vi "Autonomous Independent.vi"() -> ()   [LabVIEW 2015]
doc: "This VI is called when autonomous begins, and will automatically be terminated when autonomous ends. You can carry out timed or sensor driven robot movement independently without needing to return to the caller."
uses:
  <vilib>/Rock Robotics/Network Tables/NT Read String.vi
  <vilib>/Rock Robotics/WPI/Utilities/WPI_GetSetVariantRefNum.vi
  <vilib>/Rock Robotics/WPI/RobotDrive/WPI_RobotDriveArcadeDrive_Standard(NoSaturation).vi
  <vilib>/Rock Robotics/Network Tables/NT Write Numeric Array.vi
  <vilib>/Rock Robotics/Network Tables/NT Read Number.vi
  Robot Global Data.vi
  <vilib>/Rock Robotics/Network Tables/NT Write Boolean.vi
panel:
  out "Current Movement, for debugging":T1 {"Y Joystick Value" scale=1.0..-1.0; "X Joystick Value" scale=-1.0..1.0}
  in  "Array of robot movements":T2(array[cluster])=[{"X Joystick Value"=0.39393939393939403, "Y Joystick Value"=0.0, "Delay (sec)"=1.0, "Movement Name"="turn"}, {"X Joystick Value"=-0.3737373737373737, "Y Joystick Value"=0.0, "Delay (sec)"=1.0, "Movement Name"="turn back"}] {"Y Joystick Value" scale=1.0..-1.0; "X Joystick Value" scale=-1.0..1.0}
  # "Be sure to right-click and choose Data Operations>>Make Current Value default if you want to save the array values with the VI"
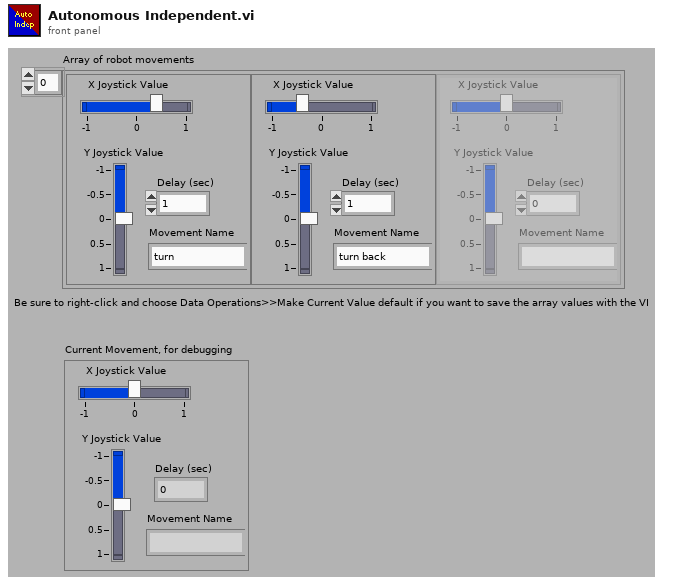
[diagram p1: front panel]
types:
  T1 = cluster{"X Joystick Value":dbl, "Y Joystick Value":dbl, "Delay (sec)":dbl, "Movement Name":string}
  T2 = cluster{"X Joystick Value":dbl, "Y Joystick Value":dbl, "Delay (sec)":dbl, "Movement Name":string}[]
  T3 = typedef "WPI_RobotDriveDevRef.ctl" = cluster{"DevStatus":errorcluster, "Motors[]":T4[], "Square Inputs":bool, "Max Output":dbl}
  T4 = typedef "WPI_MotorControlDeviceRef.ctl" = cluster{"DeviceStatus":errorcluster, "Type":T5, "PWM":cluster{"PWM Channel":T6, "DeadBand":T7}, "CAN":cluster{"Device Number":u8, "Control Mode":T8, "Semaphore":T9, "Max Vout":dbl, "TalonSRX Control Mode":T10}, "Invert":bool}
  T5 = typedef "WPI_MotorControlType.ctl" = enum16{"PWM", "CAN", "CANTalonSRX"}
  T6 = typedef "FPGA_DIOPWMChannel.ctl" = enum8{"PWM 0", "PWM 1", "PWM 2", "PWM 3", "PWM 4", "PWM 5", "PWM 6", "PWM 7", "PWM 8", "PWM 9", "PWM MXP 0", "PWM MXP 1", "PWM MXP 2", "PWM MXP 3", "PWM MXP 4", "PWM MXP 5", "PWM MXP 6", "PWM MXP 7", "PWM MXP 8", "PWM MXP 9", "Invalid"}
  T7 = typedef "WPI_PWMDeadband.ctl" = cluster{"Name":string, "maxPositivePwm":i32, "minPositivePwm":i32, "centerPwm":i32, "maxNegativePwm":i32, "minNegativePwm":i32, "angularRange":u16}
  T8 = typedef "WPI_CANJaguar_ControlMode.ctl" = enum8{"Percent VBus", "Current", "Speed", "Position", "Voltage"}
  T9 = typedef "Semaphore RefNum" = refnum<k1>
  T10 = typedef "WPI_CANTalonSRX_APIControlMode.ctl" = enum8{"Percent VBus", "Speed", "Position", "Slave", "Unchanged / Invalid", "Voltage Compensation", "Current", "Motion Profile"}
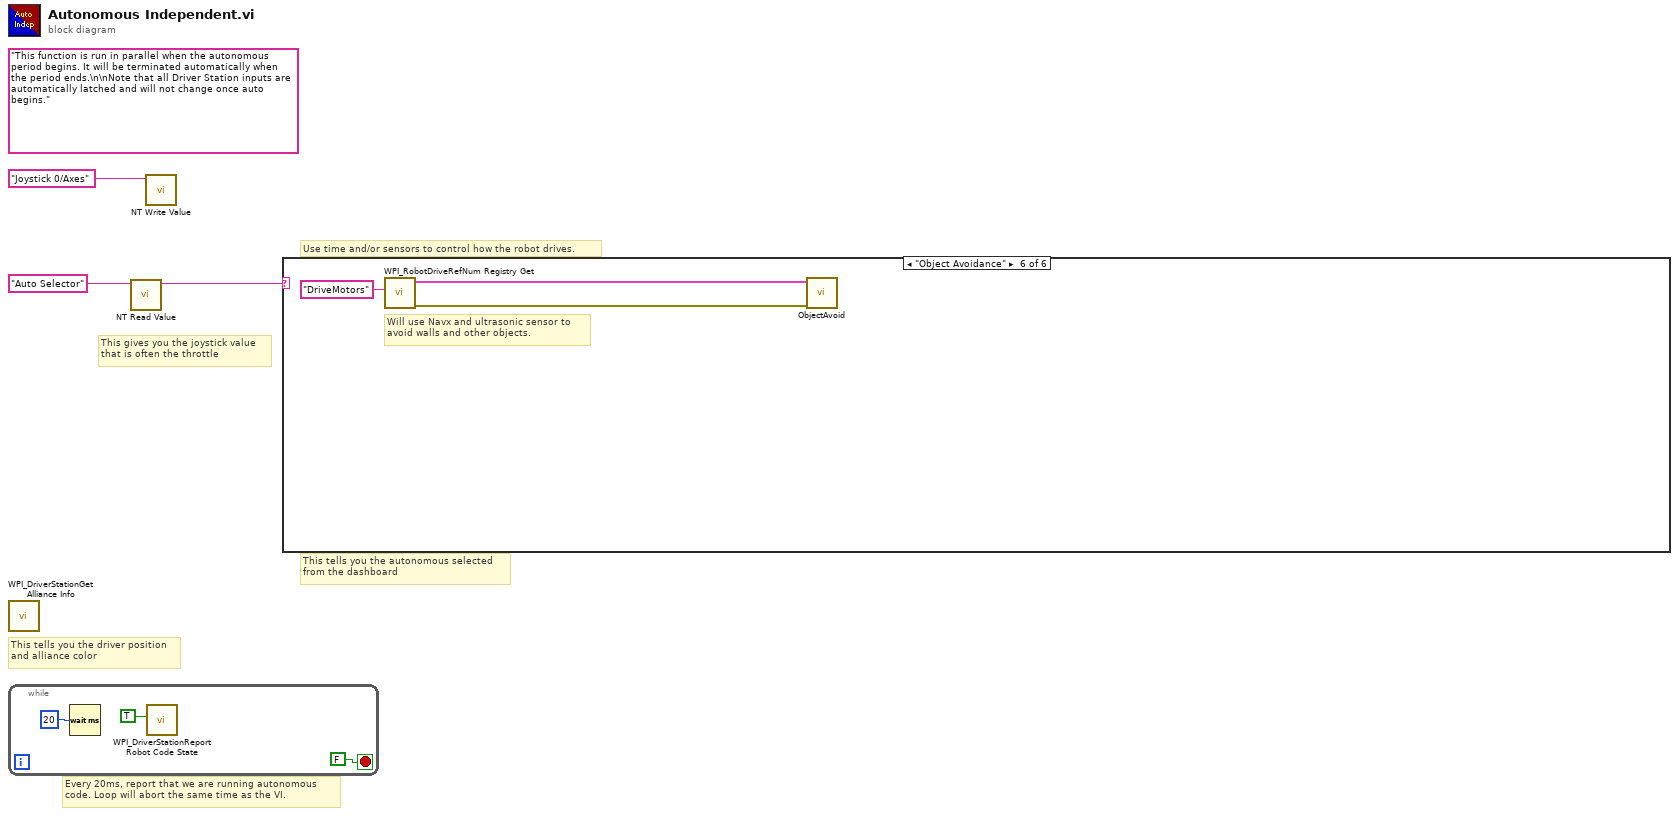
[diagram p0: block diagram]
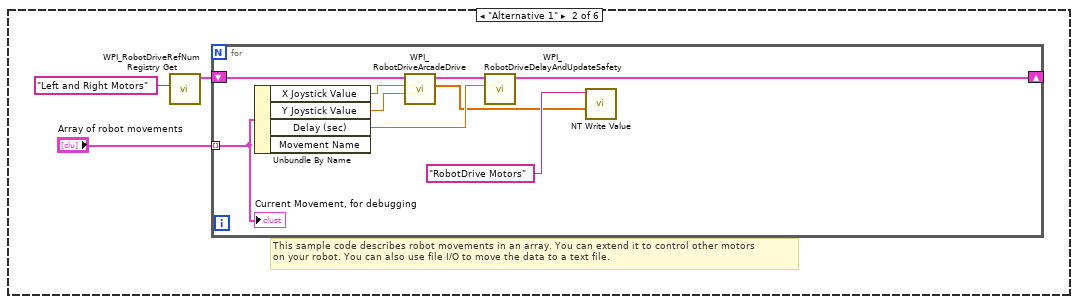
[diagram p3: hidden frame]
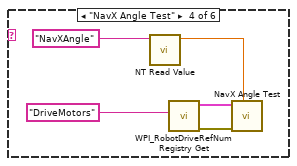
[diagram p5: hidden frame]
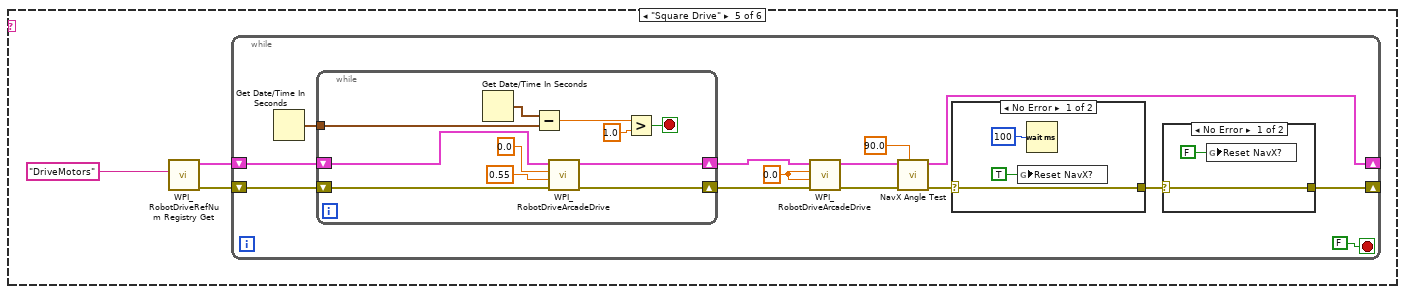
[diagram p6: hidden frame]
diagram:
  (unwired) "This function is run in parallel when the autonomous period begins. It will be terminated automatically when the period ends.\n\nNote that all Driver Station inputs are automatically latched and will not change once auto begins."
  # "This tells you the autonomous selected\nfrom the dashboard"
  # "Every 20ms, report that we are running autonomous\ncode. Loop will abort the same time as the VI."
  # "This gives you the joystick value\nthat is often the throttle"
  # "Use time and/or sensors to control how the robot drives."
  # "This tells you the driver position\nand alliance color"
  n1 = call <vilib>:"WPI_DriverStationGet Alliance Info.vi"() -> ()  [unwired: 12 out]
  n2 = while {
    stop <- FALSE stop-if-true
    n3 = Wait (ms)(milliseconds to wait=u32 20) -> ()  [unwired: 1 out]
    n4 = call <vilib>:"WPI_DriverStationReport Robot Code State.vi"("Autonomous"=TRUE) -> ()  [unwired: 10 in, 1 out]
  }
  n5 = call-poly <vilib>:"NT Read Value.vi"("Name"="Auto Selector") -> ("String"=w2:string)  [unwired: 9 in, 1 out]
  n6 = call-poly <vilib>:"NT Write Value.vi"("Name"="Joystick 0/Axes") -> ()  [unwired: 10 in, 1 out]
  n7 = case shown="\"Object Avoidance\"" w2 {
    frame Default {
      # "You can put your main auto here, or you can right-click on the case and make any\nother frame be the default case."
      # "This is the frame that will execute if no selection is made, or if it is not recognized"
    }
    frame "Alternative 1" {
      # "This sample code describes robot movements in an array. You can extend it to control other motors\non your robot. You can also use file I/O to move the data to a text file."
      n8 = call <vilib>:"WPI_RobotDriveRefNum Registry Get.vi"("refnum name"="Left and Right Motors") -> ("RobotDriveDevRef"=w8:T3)  [unwired: 1 in, 9 out]
      n9 = for {
        shift-right: [w16] -> _
        shift-left: w8 -> [w17]
        tunnel: "Array of robot movements" -> [w12] mode=indexing
        n10 = Unbundle By Name(w12) -> ("X Joystick Value"=w15:dbl, "Y Joystick Value"=w14:dbl, "Delay (sec)"=w13:dbl)  [unwired: 1 out]
        n11 = call-poly <vilib>:"WPI_RobotDriveArcadeDrive.vi"("Y axis value"=w14, "X axis value"=w15, "RobotDriveDevRef"=w17) -> ("Motor Values"=w10:dbl[], "RobotDriveDevRef"=w18:T3)  [unwired: 1 in, 6 out]
        n12 = call <vilib>:"WPI_RobotDriveDelayAndUpdateSafety.vi"("Delay (s)"=w13, "RobotDriveDevRef"=w18) -> ("RobotDriveDevRef 2"=w16:T3)  [unwired: 8 in, 1 out]
        n13 = call-poly <vilib>:"NT Write Value.vi"("Numeric Array"=w10, "Name"="RobotDrive Motors") -> ()  [unwired: 9 in, 1 out]
        "Current Movement, for debugging" <- w12
      }
    }
    frame "Alternative 2" {
      # "This is some simple sample code to drive your robot curving one direction and then the other."
    }
    frame "NavX Angle Test" {
      n14 = call-poly <vilib>:"NT Read Value.vi"("Name"="NavXAngle") -> ("Numeric"=w19:dbl)  [unwired: 9 in, 1 out]
      n15 = call <vilib>:"WPI_RobotDriveRefNum Registry Get.vi"("refnum name"="DriveMotors") -> ("error out"=w23:errorcluster, "RobotDriveDevRef"=w22:T3)  [unwired: 9 in]
      n16 = call "NavX Angle Test.vi"("Target Angle"=w19, "Error In"=w23, "RobotDriveDevRefnum"=w22) -> ()  [unwired: 6 in, 3 out]
    }
    frame "Square Drive" {
      n17 = call <vilib>:"WPI_RobotDriveRefNum Registry Get.vi"("refnum name"="DriveMotors") -> ("error out"=w24:errorcluster, "RobotDriveDevRef"=w25:T3)  [unwired: 9 in]
      n18 = while {
        shift-right: [w32] -> _
        shift-left: w25 -> [w39]
        shift-right: [w30] -> _
        shift-left: w24 -> [w40]
        stop <- FALSE stop-if-true
        w28 = 0.0 ("X axis value")
        n19 = Get Date/Time In Seconds() -> (seconds since 1Jan1904=w27:timestamp)
        n20 = while {
          shift-right: [w49] -> w38
          shift-left: w40 -> [w51]
          shift-right: [w48] -> w37
          shift-left: w39 -> [w50]
          tunnel: w27 -> [w45]
          stop <- w41 stop-if-true
          n21 = Get Date/Time In Seconds() -> (seconds since 1Jan1904=w44:timestamp)
          n22 = Subtract(x=w44, y=w45) -> (x-y=w43:dbl)
          n23 = call-poly <vilib>:"WPI_RobotDriveArcadeDrive.vi"("error in (no error)"=w51, "Y axis value"=0.55, "X axis value"=0.0, "RobotDriveDevRef"=w50) -> ("error out"=w49:errorcluster, "RobotDriveDevRef"=w48:T3)  [unwired: 5 in, 1 out]
          n24 = Greater?(x=w43, y=1.0) -> (0:w41:bool)
        }
        n25 = call-poly <vilib>:"WPI_RobotDriveArcadeDrive.vi"("error in (no error)"=w38, "Y axis value"=w28, "X axis value"=w28, "RobotDriveDevRef"=w37) -> ("error out"=w35:errorcluster, "RobotDriveDevRef"=w36:T3)  [unwired: 5 in, 1 out]
        n26 = call "NavX Angle Test.vi"("Target Angle"=90.0 ("Angle to Rotate to"), "Error In"=w35, "RobotDriveDevRefnum"=w36) -> ("error out"=w33:errorcluster, "RobotDriveDevRef"=w32:T3)  [unwired: 6 in, 1 out]
        n27 = case shown="No Error" w33 {
          selector: w33 -> [w57 w58]
          tunnel: [w57 w58] -> w31
          frame No Error {
            n28 = global write "Robot Global Data.vi" "Reset NavX?"(TRUE ("Reset NavX?")) -> ()
            n29 = Wait (ms)(milliseconds to wait=u32 100) -> ()  [unwired: 1 out]
          }
          frame Error {
          }
        }
        n30 = case shown="No Error" w31 {
          selector: w31 -> [w53 w54]
          tunnel: [w53 w54] -> w30
          frame No Error {
            n31 = global write "Robot Global Data.vi" "Reset NavX?"(FALSE ("Reset NavX?")) -> ()
          }
          frame Error {
          }
        }
      }
    }
    frame "Object Avoidance" {
      # "Will use Navx and ultrasonic sensor to \navoid walls and other objects."
      n32 = call <vilib>:"WPI_RobotDriveRefNum Registry Get.vi"("refnum name"="DriveMotors") -> ("error out"=w59:errorcluster, "RobotDriveDevRef"=w60:T3)  [unwired: 9 in]
      n33 = call "ObjectAvoid.vi"("error in (no error)"=w59, "RobotDriveDevRef"=w60) -> ()  [unwired: 9 in, 1 out]
    }
  }
